vi "采集通道设置.vi"(0 "rate":dbl=1000.0 caption="速率" format="%0.2f", 1 "sample mode":i32(ring)=10178 caption="采样模式" items=["有限采样"=10178, "连续采样"=10123, "硬件定时单点"=12522], 2 "units":i32(ring)=10348 caption="单位" items=["伏特"=10348, "来自自定义换算"=10065], 3 "number of samples per channel":i32=-1 caption="每通道采样数", 4 "input terminal configuration":i32(ring)=-1 caption="输入接线端配置" items=["默认"=-1, "RSE"=10083, "NRSE"=10078, "差分"=10106, "伪差分"=12529], 6 "physical channels":tag caption="物理通道1", 7 "physical channels 5":tag caption="物理通道5", 8 "physical channels 2":tag caption="物理通道2", 9 "physical channels 6":tag caption="物理通道6", 10 "physical channels 3":tag caption="物理通道3", 11 "physical channels 7":tag caption="物理通道7", 12 "physical channels 4":tag caption="物理通道4", 13 "physical channels 8":tag caption="物理通道8", 14 "最小采集电压值":dbl, 19 "最大采集电压值":dbl) -> (16 "波形图":waveform(dbl)[](graph))   [LabVIEW 2014]
uses:
  <vilib>/Utility/error.llb/DialogType.ctl
  <vilib>/DAQmx/read.llb/DAQmx Read (Analog 1D Wfm NChan NSamp).vi
  <vilib>/DAQmx/create/channels.llb/DAQmx Create Channel (AI-Voltage-Basic).vi
  <vilib>/DAQmx/configure/timing.llb/DAQmx Timing (Sample Clock).vi
  <vilib>/DAQmx/miscellaneous.llb/DAQmx Fill In Error Info.vi
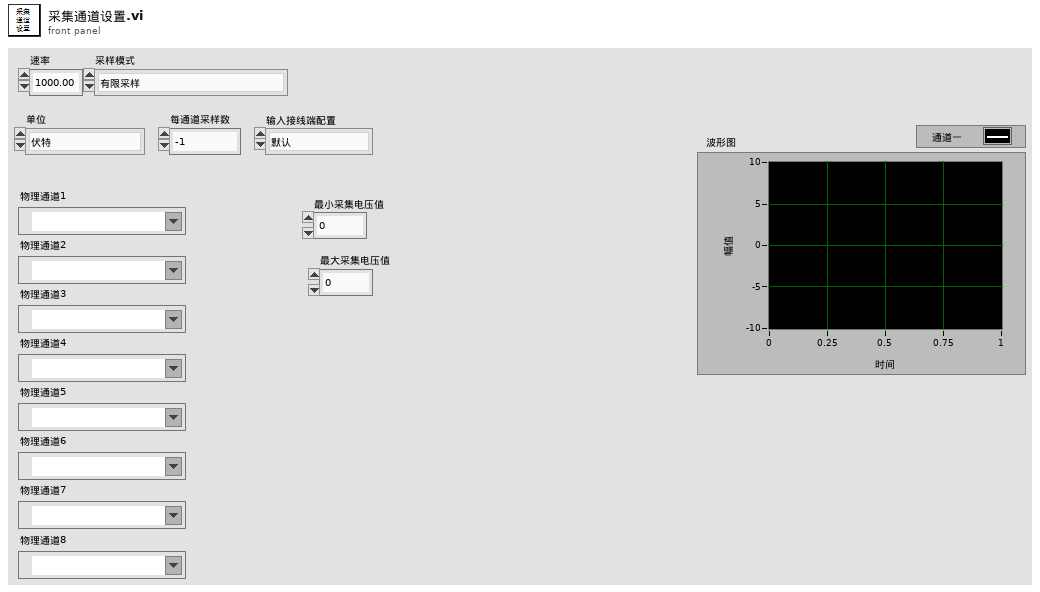
[diagram p1: front panel]
types:
  T1 = typedef "DialogType.ctl" = u16
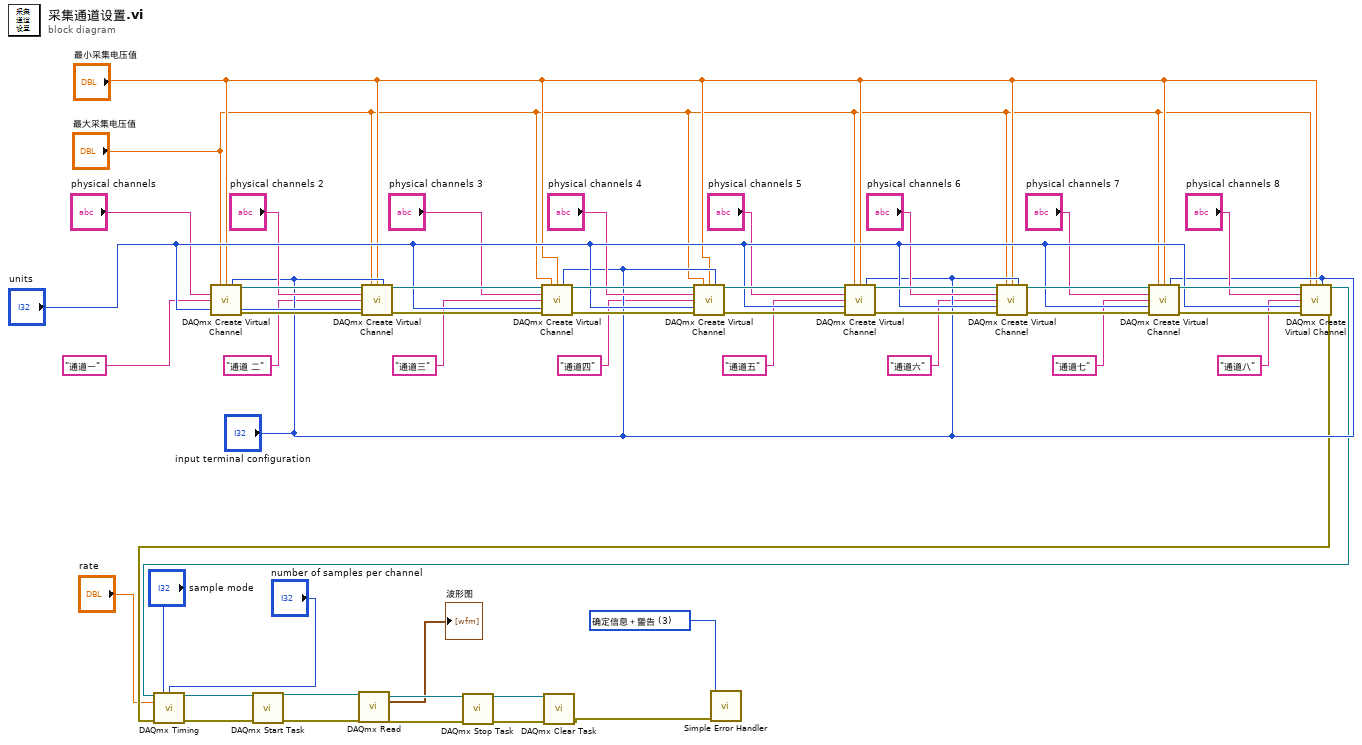
[diagram p0: block diagram]
diagram:
  w7 = T1 3 items=["无对话框", "确定信息", "继续或停止信息", "确定信息＋警告", "继续/停止+警告"] ("type of dialog (OK msg:1)")
  n1 = call-poly <vilib>:"DAQmx Create Virtual Channel.vi"("maximum value"="最大采集电压值", "minimum value"="最小采集电压值", "input terminal configuration"="input terminal configuration", "physical channels"="physical channels", "name to assign"="通道一", "units"="units") -> ("task out"=w50:refnum<k21>, "error out"=w43:errorcluster)  [unwired: 8 in]
  n2 = call-poly <vilib>:"DAQmx Create Virtual Channel.vi"("task in"=w50, "maximum value"="最大采集电压值", "minimum value"="最小采集电压值", "input terminal configuration"="input terminal configuration", "physical channels"="physical channels 2", "name to assign"="通道 二", "units"="units", "error in"=w43) -> ("task out"=w49:refnum<k21>, "error out"=w42:errorcluster)  [unwired: 6 in]
  n3 = call-poly <vilib>:"DAQmx Create Virtual Channel.vi"("task in"=w49, "maximum value"="最大采集电压值", "minimum value"="最小采集电压值", "input terminal configuration"="input terminal configuration", "physical channels"="physical channels 3", "name to assign"="通道三", "units"="units", "error in"=w42) -> ("task out"=w48:refnum<k21>, "error out"=w41:errorcluster)  [unwired: 6 in]
  n4 = call-poly <vilib>:"DAQmx Create Virtual Channel.vi"("task in"=w48, "maximum value"="最大采集电压值", "minimum value"="最小采集电压值", "input terminal configuration"="input terminal configuration", "physical channels"="physical channels 4", "name to assign"="通道四", "units"="units", "error in"=w41) -> ("task out"=w47:refnum<k21>, "error out"=w40:errorcluster)  [unwired: 6 in]
  n5 = call-poly <vilib>:"DAQmx Create Virtual Channel.vi"("task in"=w47, "maximum value"="最大采集电压值", "minimum value"="最小采集电压值", "input terminal configuration"="input terminal configuration", "physical channels"="physical channels 5", "name to assign"="通道五", "units"="units", "error in"=w40) -> ("task out"=w46:refnum<k21>, "error out"=w39:errorcluster)  [unwired: 6 in]
  n6 = call-poly <vilib>:"DAQmx Create Virtual Channel.vi"("task in"=w46, "maximum value"="最大采集电压值", "minimum value"="最小采集电压值", "input terminal configuration"="input terminal configuration", "physical channels"="physical channels 6", "name to assign"="通道六", "units"="units", "error in"=w39) -> ("task out"=w45:refnum<k21>, "error out"=w38:errorcluster)  [unwired: 6 in]
  n7 = call-poly <vilib>:"DAQmx Create Virtual Channel.vi"("task in"=w45, "maximum value"="最大采集电压值", "minimum value"="最小采集电压值", "input terminal configuration"="input terminal configuration", "physical channels"="physical channels 7", "name to assign"="通道七", "units"="units", "error in"=w38) -> ("task out"=w44:refnum<k21>, "error out"=w37:errorcluster)  [unwired: 6 in]
  n8 = call-poly <vilib>:"DAQmx Create Virtual Channel.vi"("task in"=w44, "maximum value"="最大采集电压值", "minimum value"="最小采集电压值", "input terminal configuration"="input terminal configuration", "physical channels"="physical channels 8", "name to assign"="通道八", "units"="units", "error in"=w37) -> ("task out"=w18:refnum<k21>, "error out"=w17:errorcluster)  [unwired: 6 in]
  n9 = call-poly <vilib>:"DAQmx Timing.vi"("task/channels in"=w18, "sample mode"="sample mode", "samples per channel"="number of samples per channel", "rate"="rate", "error in"=w17) -> ("task out"=w15:refnum<k21>, "error out"=w14:errorcluster)  [unwired: 9 in]
  n10 = call <vilib>:"DAQmx Start Task.vi"("task/channels in"=w15, "error in"=w14) -> ("task out"=w13:refnum<k21>, "error out"=w12:errorcluster)  [unwired: 12 in]
  n11 = call-poly <vilib>:"DAQmx Read.vi"("task/channels in"=w13, "error in"=w12) -> ("task out"=w11:refnum<k21>, "data"=→"波形图":waveform(dbl)[], "error out"=w10:errorcluster)  [unwired: 11 in]
  n12 = call <vilib>:"DAQmx Stop Task.vi"("task/channels in"=w11, "error in"=w10) -> ("task out"=w9:refnum<k21>, "error out"=w8:errorcluster)  [unwired: 12 in]
  n13 = call <vilib>:"DAQmx Clear Task.vi"("task in"=w9, "error in"=w8) -> ("error out"=w6:errorcluster)  [unwired: 13 in]
  n14 = call <vilib>:"Simple Error Handler.vi"("type of dialog (OK msg:1)"=w7, "error in (no error)"=w6) -> ()  [unwired: 3 in, 5 out]
